vi "Read Value Source.vi"(8 "error in (no error)":errorcluster, 11 "Composed Column in":refnum<class "Composed Column.lvclass">) -> (0 "error out":errorcluster, 2 "Value Source":refnum<class "Value Source.lvclass">, 3 "Composed Column out":refnum<class "Composed Column.lvclass">)   [LabVIEW 2020, in "Composed Columns.lvlib" / "Composed Column.lvclass"]
uses:
  Composed Column.lvclass
  Composed Columns/Value Source Interface Class/Value Source.lvclass
  Composed Column.lvclass/Composed Column.ctl
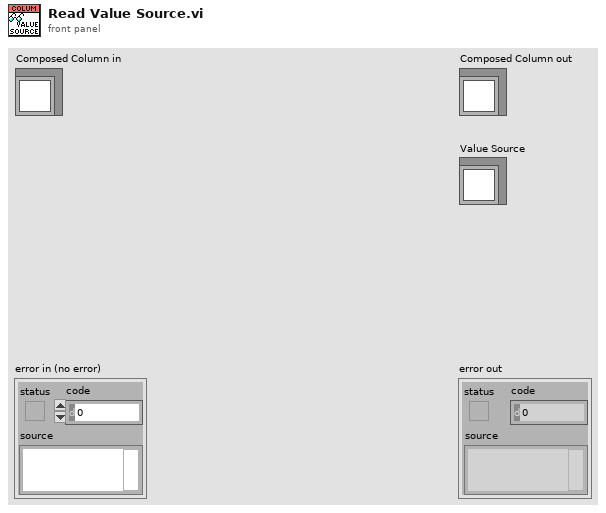
[diagram p1: front panel]
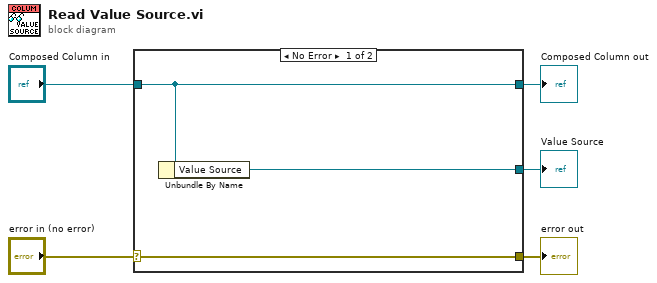
[diagram p0: block diagram]
diagram:
  n1 = case shown="No Error" "error in (no error)" {
    selector: "error in (no error)" -> [w8 w9]
    tunnel: [w8 w9] -> w4
    tunnel: [w7 w10] -> w2
    tunnel: "Composed Column in" -> [w7 w10]
    tunnel: [w6 _] -> w1
    frame No Error {
      n2 = Unbundle By Name(w7) -> ("Value Source"=w6:refnum<class "Value Source.lvclass">)
    }
    frame Error {
    }
  }
  "error out" <- w4
  "Composed Column out" <- w2
  "Value Source" <- w1
